vi "Release-message-queues.vi"(8 "error in (no error)":errorcluster, 11 "Object ref in":T1) -> (0 "error out":errorcluster, 3 "Object ref out":T1)   [LabVIEW 2013, in "SLMControl.lvlib" / "SC-Main.lvclass"]
uses:
  SC-Main.lvclass
  Object-reference.ctl
  SC-Main.lvclass/SC-Main.ctl
  Read Action queue.vi
  Read Deposition queue.vi
  Read Lasing queue.vi
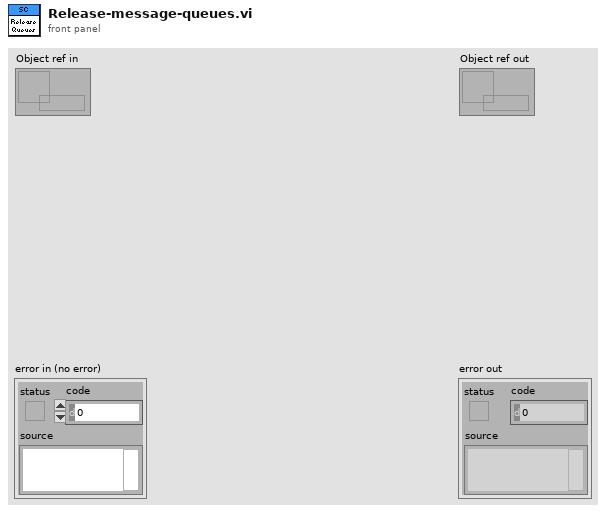
[diagram p1: front panel]
types:
  T1 = typedef "SLMControl.lvlib/SC-Main.lvclass/Object-reference.ctl" = refnum<data-value>
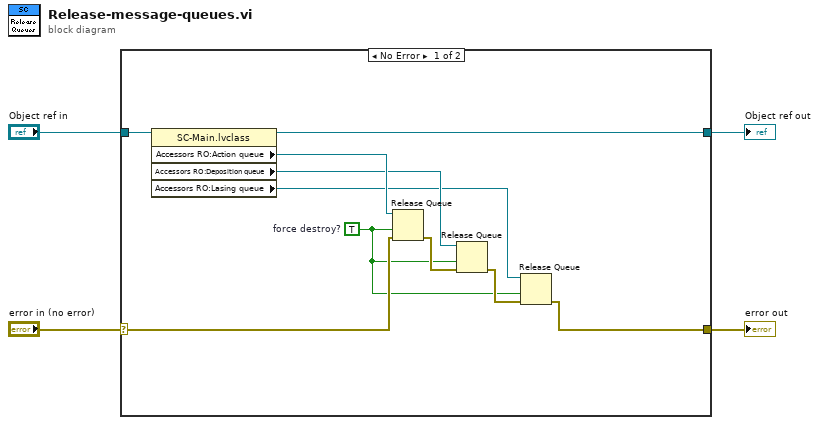
[diagram p0: block diagram]
diagram:
  n1 = case shown="No Error" "error in (no error)" {
    selector: "error in (no error)" -> [w11 w16]
    tunnel: [w7 w16] -> w3
    tunnel: [w13 w15] -> w1
    tunnel: "Object ref in" -> [w14 w15]
    frame No Error {
      w5 = TRUE  # force destroy?
      n2 = property class="SC-Main.lvclass"(reference=w14) -> (reference out=w13:T1, "Accessors RO:Action queue"=w12:refnum<queue>, "Accessors RO:Deposition queue"=w10:refnum<queue>, "Accessors RO:Lasing queue"=w6:refnum<queue>)  [unwired: 1 in, 1 out]
      n3 = Release Queue(queue=w12, force destroy? (F)=w5, error in (no error)=w11) -> (error out=w9:errorcluster)  [unwired: 2 out]
      n4 = Release Queue(queue=w10, force destroy? (F)=w5, error in (no error)=w9) -> (error out=w8:errorcluster)  [unwired: 2 out]
      n5 = Release Queue(queue=w6, force destroy? (F)=w5, error in (no error)=w8) -> (error out=w7:errorcluster)  [unwired: 2 out]
    }
    frame Error {
    }
  }
  "error out" <- w3
  "Object ref out" <- w1
